vi "Run WriteUR Core.vi"(8 "error in (no error)":errorcluster, 11 "MB in":refnum<class "Master CR.lvclass">) -> (0 "error out":errorcluster)   [LabVIEW 2021, in "Master CR.lvclass"]
uses:
  Master CR.lvclass
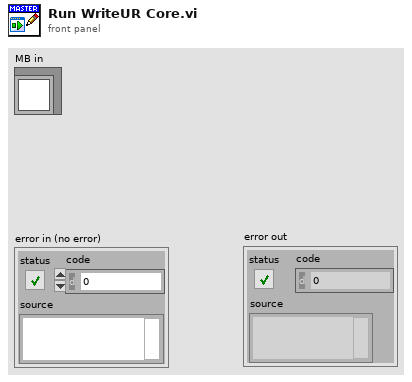
[diagram p1: front panel]
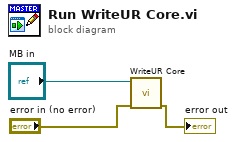
[diagram p0: block diagram]
diagram:
  n1 = call-dynamic "WriteUR Core.vi"("error in (no error)"="error in (no error)", "Master CR in"="MB in") -> ("error out"=→"error out":errorcluster)  [unwired: 9 in]
